vi "Error to json and back.vi"() -> ()   [LabVIEW 2026]
uses:
  <vilib>/MultiError/TokenizeJSON/Multi Error Cluster.lvlib
panel:
  in  "s":bool
  out "size(s)":i32
  out "error out 2":errorcluster
  out "array of errors":errorcluster[](array[cluster])
  out "source":string
  out "error out":errorcluster
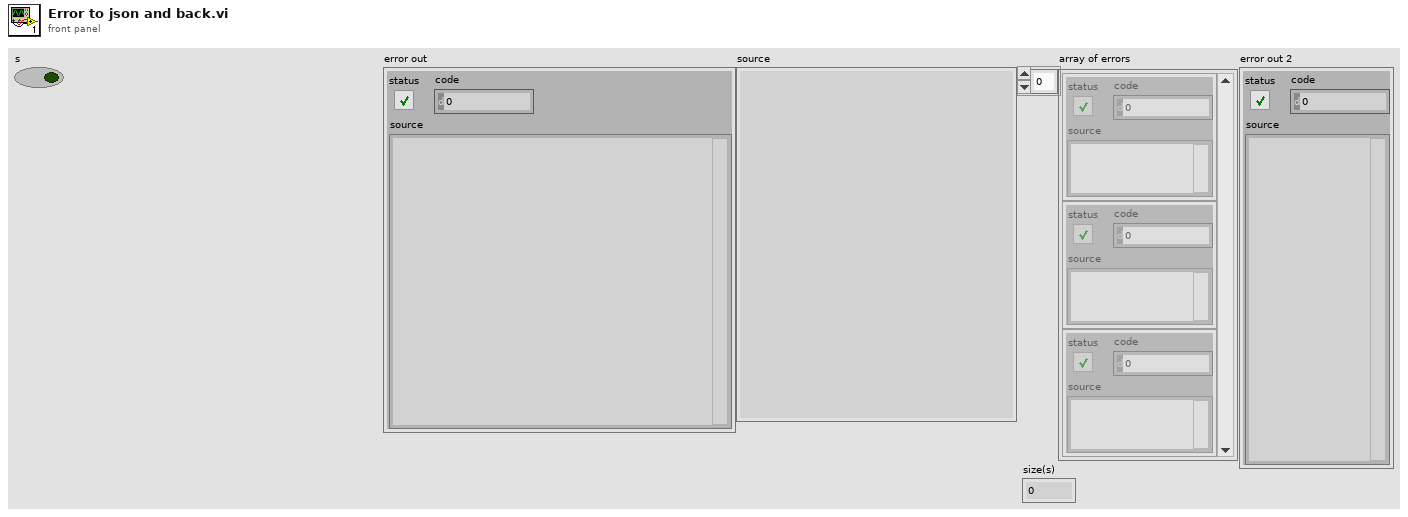
[diagram p1: front panel]
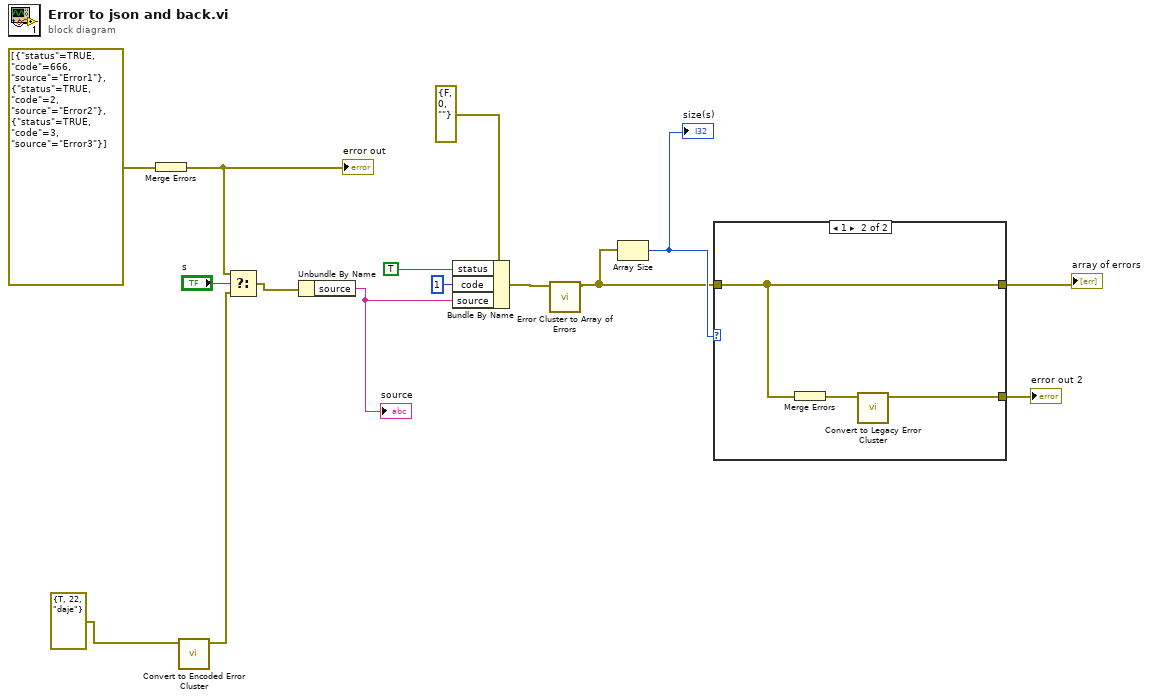
[diagram p0: block diagram]
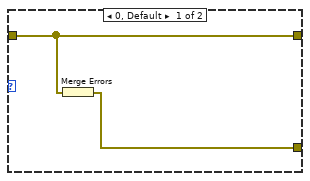
[diagram p2: hidden frame]
diagram:
  n1 = Merge Errors(errorcluster[] [{"status"=TRUE, "code"=666, "source"="Error1"}, {"status"=TRUE, "code"=2, "source"="Error2"}, {"status"=TRUE, "code"=3, "source"="Error3"}] ("error constant")) -> (w3:errorcluster)
  "error out" <- w3
  n2 = call <vilib>:"Convert to Encoded Error Cluster.vi"("error in"=errorcluster {"status"=TRUE, "code"=22, "source"="daje"}) -> ("error out"=w4:errorcluster)  [unwired: 10 in]
  n3 = Select(t=w3, s="s", f=w4) -> (s? t:f=w2:errorcluster)
  n4 = Unbundle By Name(w2) -> ("source"=w11:string)
  "source" <- w11
  n5 = Bundle By Name(cluster=errorcluster {"status"=FALSE, "code"=0, "source"=""} ("error constant"), "status"=TRUE, "code"=1, "source"=w11) -> (w10:errorcluster)
  n6 = call <vilib>:"Error Cluster to Array of Errors.vi"("error"=w10) -> ("array of errors"=w5:errorcluster[])  [unwired: 10 in]
  n7 = Array Size(array=w5) -> (size(s)=w6:i32)
  "size(s)" <- w6
  n8 = case shown="1" w6 {
    tunnel: [w16 w18] -> w9
    tunnel: w5 -> [w17 w19]
    tunnel: [w17 w19] -> w7
    frame 0, Default {
      n9 = Merge Errors(w17) -> (w16:errorcluster)
    }
    frame 1 {
      n10 = Merge Errors(w19) -> (w20:errorcluster)
      n11 = call <vilib>:"Convert to Legacy Error Cluster.vi"("error in"=w20) -> ("error out"=w18:errorcluster)  [unwired: 10 in]
    }
  }
  "array of errors" <- w7
  "error out 2" <- w9
